vi "Set PID.vi"(8 "error in (no error)":errorcluster, 10 "Control Parameters":cluster{"P":dbl, "I":dbl, "D":u16}, 11 "Lakeshore 331 in":refnum<class "Lakeshore 331.lvclass">) -> (0 "error out":errorcluster, 3 "Lakeshore 331 out":refnum<class "Lakeshore 331.lvclass">)   [LabVIEW 2022 SP3, in "Lakeshore 331.lvclass"]
uses:
  Lakeshore 331.lvclass
  Lakeshore 331.lvclass/Lakeshore 331.ctl
  Temp Control.lvclass
  <instrlib>/Lake Shore Cryotronics 331/Lake Shore Cryotronics 331.lvlib
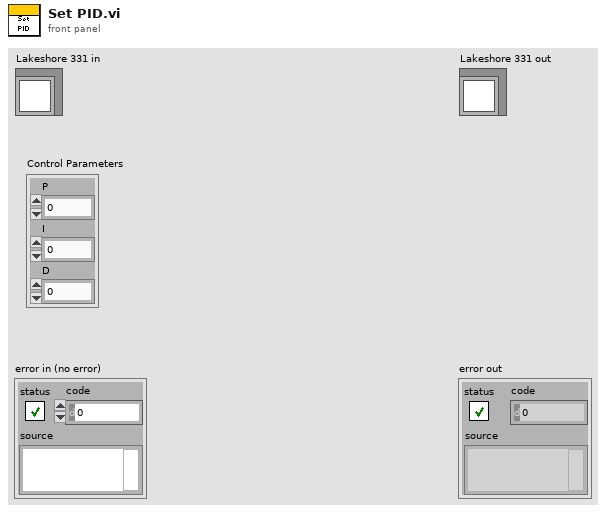
[diagram p1: front panel]
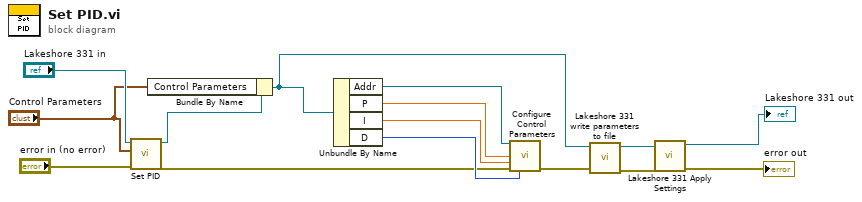
[diagram p0: block diagram]
diagram:
  n1 = call-parent "Set PID.vi"("error in (no error)"="error in (no error)", "Control Parameters"="Control Parameters", "Temp Control in"="Lakeshore 331 in") -> ("error out"=w9:errorcluster, "Temp Control out"=w8:refnum<class "Lakeshore 331.lvclass">)  [unwired: 7 in]
  n2 = Bundle By Name(cluster=w8, "Control Parameters"="Control Parameters") -> (w5:refnum<class "Lakeshore 331.lvclass">)
  n3 = Unbundle By Name(w5) -> ("Addr"=w13:refnum<visa-resource-name>, "P"=w12:dbl, "I"=w11:dbl, "D"=w10:u16)
  n4 = call <instrlib>:"Configure Control Parameters.vi"("VISA resource name"=w13, "Gain (P) (0.0)"=w12, "Reset (I) (0.0)"=w11, "error in (no error)"=w9, "Rate (D) (0)"=w10) -> ("error out"=w6:errorcluster)  [unwired: 9 in, 1 out]
  n5 = call "Lakeshore 331 write parameters to file.vi"("error in (no error)"=w6, "Lakeshore 331 in"=w5) -> ("error out"=w4:errorcluster, "Lakeshore 331 out"=w3:refnum<class "Lakeshore 331.lvclass">)  [unwired: 8 in]
  n6 = call "Lakeshore 331 Apply Settings.vi"("error in (no error)"=w4, "Lakeshore 331 in"=w3) -> ("error out"=→"error out":errorcluster, "Lakeshore 331 out"=→"Lakeshore 331 out":refnum<class "Lakeshore 331.lvclass">)  [unwired: 8 in]
